vi "PH_PSDBController.PC get PSDB Information.vi"(0 "i ref in":refnum<vi>, 5 "error IO":errorcluster) -> (14 "i ref out":refnum<vi>, 19 "error out":errorcluster)   [LabVIEW 2014, in "PH_PSDBController.lvlib"]
doc: "Within this VI the process event to ask the data base for available shot types and experiments is handeled."
uses:
  PH_PSDBController.lvlib
  PH_PSDBWriter/PH_PSDBWriter.Data Status.ctl
  User/Eisenbarth/psdb_lv/PSDB.lvlib
  PH_PSDBWriter/PH_PSDBWriter.lvlib
  PH_Common/PH_Common.lvlib
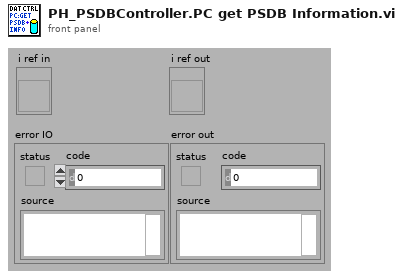
[diagram p1: front panel]
types:
  T1 = typedef "PH_PSDBWriter.lvlib/PH_PSDBWriter.Data Status.ctl" = i16
  T2 = typedef "PH_PSDBController.lvlib/PH_PSDBController.i attribute.ctl" = cluster{"GUI Refs":cluster{"Data Status":refnum<vi>, "Current Shot ID":refnum<vi>, "active Subsystems":refnum<vi>, "Experiment Description":refnum<vi>, "Shot Comment":refnum<vi>, "Experiment":refnum<vi>, "Shottype":refnum<vi>, "Sequencer SM State":refnum<vi>, "Instances with Errors":refnum<vi>}, "Service ID Shot ID":i32, "Service ID wanted Subsystem":i32, "Data Status":T1, "Shotinformation":cluster{"Current Experiment ID":i32, "Current Shot Type":i32, "Current Comment":string}, "Data taking?":bool, "Service ID current Shottype":i32, "Service ID current Experiment":i32, "Service ID currentShot Comment":i32, "Service ID possible Shottypes":i32, "Service ID possible Experiments":i32, "possible Experiments":T3[], "possible Shottypes":T3[], "List":cluster{"Info":cluster{"Instance":string, "Data Status":T1}[], "GUI Ref":refnum<vi>, "Classname":string}[], "Subsystems Off?":cluster{"PHELIX_Beamline_fs_YLF_BL_Status":bool, "PHELIX_Beamline_ns_BL_Status":bool, "PHELIX_Beamline_PA_Input_BL_Status":bool, "PHELIX_Beamline_PA_MA_BL_Status":bool, "PHELIX_Beamline_MA_Z6_BL_Status":bool, "PHELIX_Beamline_MA_LB_BL_Status":bool, "PHELIX_Beamline_PA_LL_BL_Status":bool}, "PSDB Credentials":T4}
  T3 = typedef "PSDB.lvlib/PSDB_Info.ctl" = cluster{"Name":string, "Description":string, "ID":i32}
  T4 = typedef "PH_Common.lvlib/PH_Connection.PSDB Credentials.ctl" = cluster{"PW":string, "ID":string, "DS":string}
  T5 = typedef "NI_Database_API.lvlib/Conn ObjectReference.ctl" = refnum<k1>
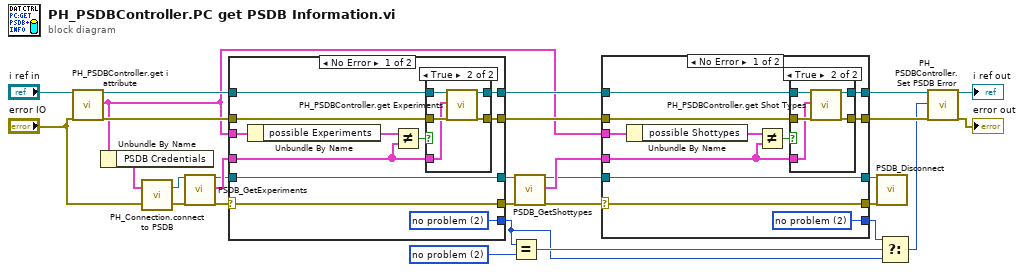
[diagram p0: block diagram]
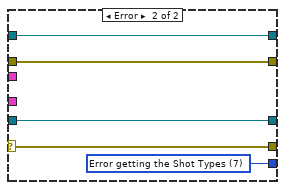
[diagram p3: hidden frame]
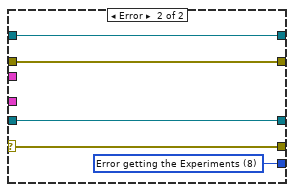
[diagram p5: hidden frame]
diagram:
  w10 = T1 2 items=["no info", "no Data collection", "no problem", "Error getting the instance ID", "Error writing Data to data base", "Error concerning the subsystem", "Error getting the Shot ID", "Error getting the Shot Types", "Error getting the Experiments"] ("Data Status")
  n1 = call "PH_PSDBController.get i attribute.vi"("i ref in"="i ref in", "error in (no error)"="error IO") -> ("i ref out"=w26:refnum<vi>, "i attribute"=w2:T2, "error out"=w5:errorcluster)  [unwired: 15 in]
  n2 = Unbundle By Name(w2) -> ("PSDB Credentials"=w1:T4)
  n3 = call "PH_Connection.connect to PSDB.vi"("error in"="error IO", "PSDB Credentials"=w1) -> ("error out"=w28:errorcluster, "connection reference"=w29:T5)
  n4 = call "PSDB_GetExperiments.vi"("connection reference"=w29, "error in (no error)"=w28) -> ("connection reference out"=w23:T5, "Experiments"=w27:T3[], "error out"=w25:errorcluster)  [unwired: 15 in]
  n5 = case shown="No Error" w25 {
    selector: w25 -> [w32 w52]
    tunnel: w27 -> [w35 _]
    tunnel: w2 -> [w40 _]
    tunnel: w26 -> [w38 w50]
    tunnel: [w37 w50] -> w20
    tunnel: [w36 w49] -> w19
    tunnel: w5 -> [w33 w49]
    tunnel: [w32 w52] -> w24
    tunnel: w23 -> [w31 w51]
    tunnel: [w31 w51] -> w22
    tunnel: [w30 w48] -> w6
    frame No Error {
      w30 = T1 2 items=["no info", "no Data collection", "no problem", "Error getting the instance ID", "Error writing Data to data base", "Error concerning the subsystem", "Error getting the Shot ID", "Error getting the Shot Types", "Error getting the Experiments"] ("Data Status")
      n6 = Unbundle By Name(w40) -> ("possible Experiments"=w39:T3[])
      n7 = Not Equal?(x=w39, y=w35) -> (x != y?=w34:bool)
      n8 = case shown="True" w34 {
        tunnel: w33 -> [w41 w47]
        tunnel: w38 -> [w42 w46]
        tunnel: [w42 w44] -> w37
        tunnel: [w41 w43] -> w36
        tunnel: w35 -> [_ w45]
        frame False {
        }
        frame True {
          n9 = call "PH_PSDBController.get Experiments.vi"("i ref in"=w46, "possible Experiments"=w45, "error IO"=w47) -> ("i ref out"=w44:refnum<vi>, "error out"=w43:errorcluster)  [unwired: 15 in]
        }
      }
    }
    frame Error {
      w48 = T1 8 items=["no info", "no Data collection", "no problem", "Error getting the instance ID", "Error writing Data to data base", "Error concerning the subsystem", "Error getting the Shot ID", "Error getting the Shot Types", "Error getting the Experiments"] ("Data Status")
    }
  }
  n10 = Equal?(x=w6, y=w10) -> (x = y?=w9:bool)
  n11 = call "PSDB_GetShottypes.vi"("connection reference"=w22, "error in (no error)"=w24) -> ("connection reference out"=w17:T5, "Shottypes"=w21:T3[], "error out"=w18:errorcluster)  [unwired: 15 in]
  n12 = case shown="No Error" w18 {
    selector: w18 -> [w55 w75]
    tunnel: w21 -> [w58 _]
    tunnel: w2 -> [w63 _]
    tunnel: w20 -> [w61 w72]
    tunnel: [w60 w72] -> w13
    tunnel: [w59 w71] -> w11
    tunnel: w19 -> [w56 w71]
    tunnel: [w55 w75] -> w15
    tunnel: w17 -> [w54 w74]
    tunnel: [w54 w74] -> w16
    tunnel: [w53 w73] -> w8
    frame No Error {
      w53 = T1 2 items=["no info", "no Data collection", "no problem", "Error getting the instance ID", "Error writing Data to data base", "Error concerning the subsystem", "Error getting the Shot ID", "Error getting the Shot Types", "Error getting the Experiments"] ("Data Status")
      n13 = Unbundle By Name(w63) -> ("possible Shottypes"=w62:T3[])
      n14 = Not Equal?(x=w62, y=w58) -> (x != y?=w57:bool)
      n15 = case shown="True" w57 {
        tunnel: w56 -> [w64 w70]
        tunnel: w61 -> [w65 w69]
        tunnel: [w65 w67] -> w60
        tunnel: [w64 w66] -> w59
        tunnel: w58 -> [_ w68]
        frame False {
        }
        frame True {
          n16 = call "PH_PSDBController.get Shot Types.vi"("i ref in"=w69, "possible Shot Types"=w68, "error IO"=w70) -> ("i ref out"=w67:refnum<vi>, "error out"=w66:errorcluster)  [unwired: 15 in]
        }
      }
    }
    frame Error {
      w73 = T1 7 items=["no info", "no Data collection", "no problem", "Error getting the instance ID", "Error writing Data to data base", "Error concerning the subsystem", "Error getting the Shot ID", "Error getting the Shot Types", "Error getting the Experiments"] ("Data Status")
    }
  }
  n17 = call "PSDB_Disconnect.vi"("connection reference"=w16, "error in (no error)"=w15) -> ()  [unwired: 17 in, 1 out]
  n18 = Select(t=w8, s=w9, f=w6) -> (s? t:f=w7:T1)
  n19 = call "PH_PSDBController.Set PSDB Error.vi"("i ref in"=w13, "Data Status"=w7, "error in"=w11) -> ("i ref out"=→"i ref out":refnum<vi>, "error out"=→"error out":errorcluster)  [unwired: 15 in]
